vi "Senden_ECD.vi"(5 "error in":errorcluster, 6 "BefehlsCluster":T1, 7 "AbfragenCluster":cluster{string[], string[], string[]}, 8 "Abfragenr.Cluster":cluster{i32, i32, i32}, 9 "Senden?":bool[](array[boolean]), 10 "FPGA-VI-Referenz":refnum<k20>) -> (0 "BefehlsCluster":T1, 2 "error out":errorcluster, 3 "Senden?":bool[](array[boolean]), 4 "Abfragenr.Cluster":cluster{i32, i32, i32})   [LabVIEW 2017]
uses:
  <vilib>/Utility/error.llb/Error Cluster From Error Code.vi
  <vilib>/rvi/errors/niLvFpgaAdjustHostInterfaceError.vi
  <vilib>/rvi/interface/nirviMethod/nirviMethod.xnode
  FPGA Bitfiles/HAGAR-VECD_FPGATarget_FPGA-ProgrammECD_WS++LmW9gGg.lvbitx
  FPGA-Programm_ECD.vi
  <vilib>/rvi/errors/niLvFpgaMergeErrorWithErrorCode.vi
  <vilib>/FPGAPlugInAG/cRIO-9035/niLvFpga_WriteFifo_cRIO-9035.vi
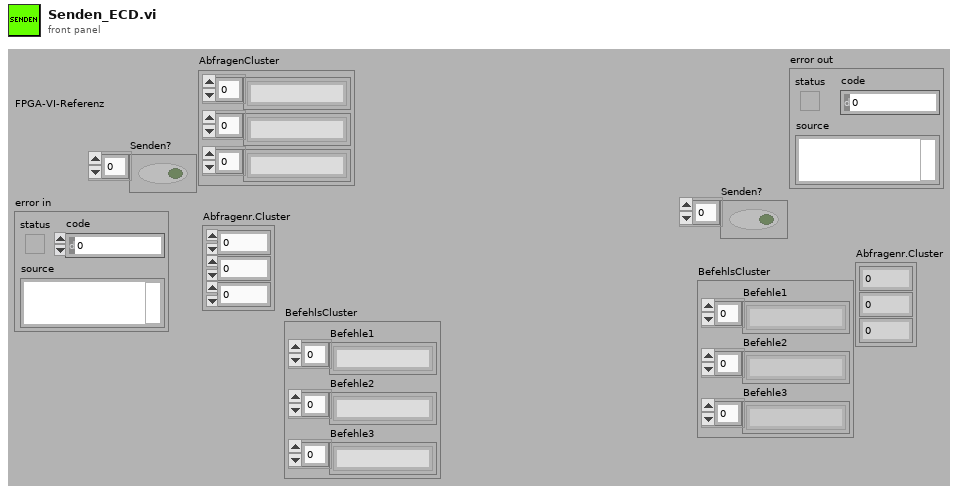
[diagram p1: front panel]
types:
  T1 = cluster{"Befehle1":string[], "Befehle2":string[], "Befehle3":string[]}
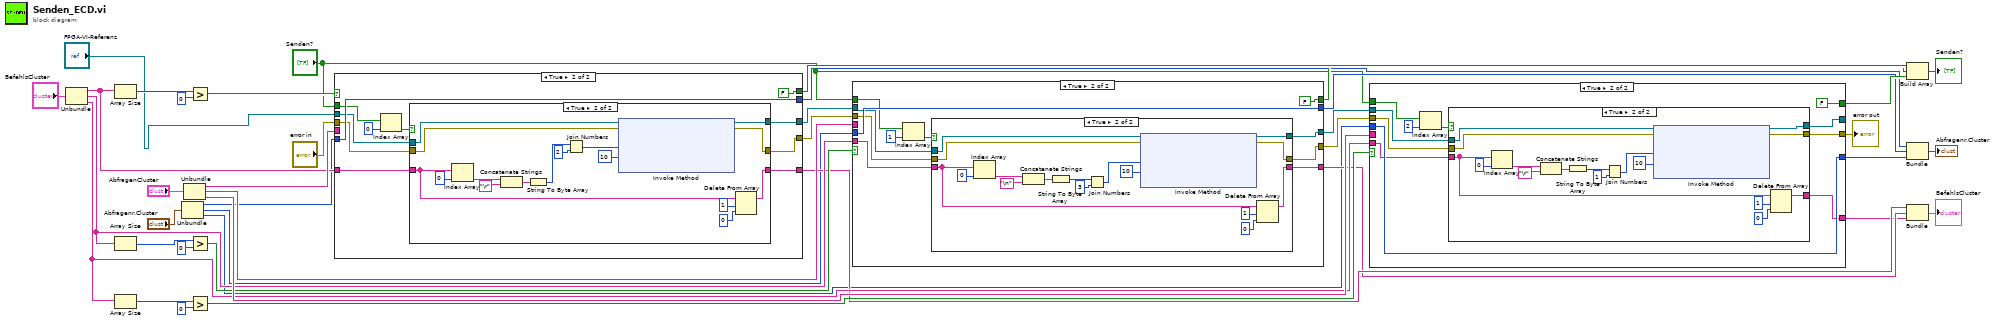
[diagram p0: block diagram]
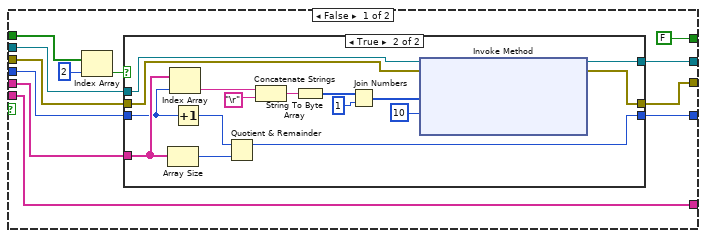
[diagram p2: hidden frame]
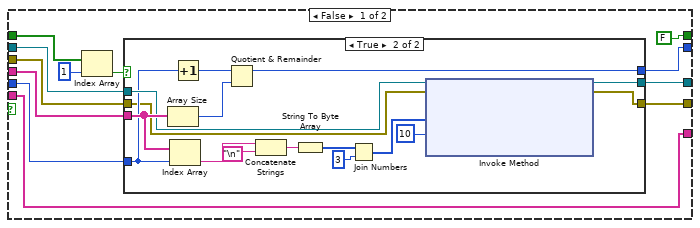
[diagram p5: hidden frame]
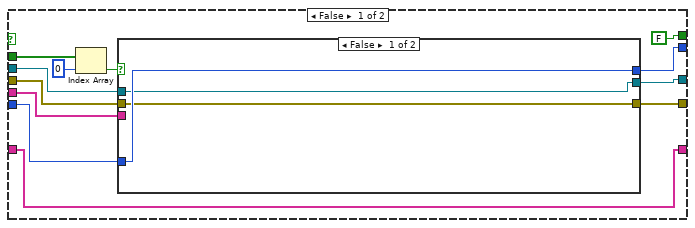
[diagram p8: hidden frame]
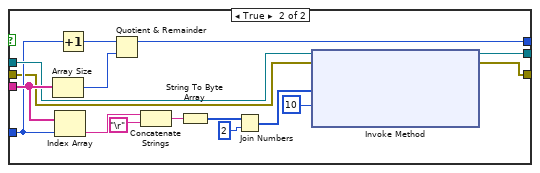
[diagram p9: hidden frame]
diagram:
  n1 = Unbundle("BefehlsCluster") -> ("Befehle1"=w26:string[], "Befehle2"=w25:string[], "Befehle3"=w24:string[])
  n2 = Array Size(array=w26) -> (size(s)=w41:i32)
  n3 = Array Size(array=w25) -> (size(s)=w35:i32)
  n4 = Array Size(array=w24) -> (size(s)=w32:i32)
  n5 = Unbundle("Abfragenr.Cluster") -> (w14:i32, w13:i32, w12:i32)
  n6 = Unbundle("AbfragenCluster") -> (w38:string[], w37:string[], w36:string[])
  n7 = Greater?(x=w41, y=0) -> (0:w39:bool)
  n8 = Greater?(x=w35, y=0) -> (0:w33:bool)
  n9 = Greater?(x=w32, y=0) -> (0:w30:bool)
  n10 = case shown="True" w39 {
    tunnel: w26 -> [w53 w80]
    tunnel: [w53 w79] -> w23
    tunnel: "Senden?" -> [w47 w77]
    tunnel: [FALSE FALSE] -> w19
    tunnel: w14 -> [w50 w83]
    tunnel: "FPGA-VI-Referenz" -> [w49 w78]
    tunnel: [w48 w83] -> w11
    tunnel: w38 -> [w46 _]
    tunnel: [w45 w76] -> w29
    tunnel: "error in" -> [w43 w74]
    tunnel: [w42 w73] -> w4
    frame False {
      n11 = Index Array(array=w47, index=0 ("Index")) -> (element=w51:bool)
      n12 = case shown="False" w51 {
        tunnel: w46 -> [_ w70]
        tunnel: w50 -> [w56 w64]
        tunnel: w49 -> [w55 w67]
        tunnel: [w56 w63] -> w48
        tunnel: [w55 w62] -> w45
        tunnel: w43 -> [w54 w58]
        tunnel: [w54 w57] -> w42
        frame False {
        }
        frame True {
          n13 = Array Size(array=w70) -> (size(s)=w71:i32)
          n14 = Index Array(array=w70, index=w64) -> (element=w60:string)
          n15 = Increment(x=w64) -> (x+1=w72:i32)
          n16 = Quotient & Remainder(x=w72, y=w71) -> (x-y*floor(x/y)=w63:i32)  [unwired: 1 out]
          n17 = Concatenate Strings(w60, "\r") -> (w61:string)
          n18 = String To Byte Array(string=w61) -> (unsigned byte array=w69:u8[])
          n19 = Join Numbers(hi=w69, lo=u8 2) -> ((hi.lo)=w66:u16[])
          n20 = xnode "Invoke Method"("FPGA-VI-Referenz (Eingang)"=w67, "Fehler (Eingang)"=w58, "Daten"=w66, "Timeout (ms)"=10) -> ("FPGA-VI-Referenz (Ausgang)"=w62:refnum<k20>, "Fehler (Ausgang)"=w57:errorcluster)  [unwired: 1 out]
        }
      }
    }
    frame True {
      n21 = Index Array(array=w77, index=0 ("Index")) -> (element=w81:bool)
      n22 = case shown="True" w81 {
        tunnel: w80 -> [w86 w98]
        tunnel: [w86 w100] -> w79
        tunnel: w78 -> [w85 w99]
        tunnel: [w85 w92] -> w76
        tunnel: w74 -> [w84 w88]
        tunnel: [w84 w87] -> w73
        frame False {
        }
        frame True {
          n23 = Index Array(array=w98, index=0 ("Index")) -> (element=w90:string)
          n24 = Concatenate Strings(w90, "\r") -> (w89:string)
          n25 = String To Byte Array(string=w89) -> (unsigned byte array=w96:u8[])
          n26 = Join Numbers(hi=w96, lo=u8 2) -> ((hi.lo)=w94:u16[])
          n27 = xnode "Invoke Method"("FPGA-VI-Referenz (Eingang)"=w99, "Fehler (Eingang)"=w88, "Daten"=w94, "Timeout (ms)"=10) -> ("FPGA-VI-Referenz (Ausgang)"=w92:refnum<k20>, "Fehler (Ausgang)"=w87:errorcluster)  [unwired: 1 out]
          n28 = Delete From Array(array=w98, length=1 ("Länge"), index=0 ("Index")) -> (array with subset deleted=w100:string[])  [unwired: 1 out]
        }
      }
    }
  }
  n29 = case shown="True" w33 {
    tunnel: w25 -> [w114 w141]
    tunnel: [w114 w140] -> w22
    tunnel: "Senden?" -> [w108 w138]
    tunnel: w13 -> [w111 w144]
    tunnel: w29 -> [w110 w139]
    tunnel: [w109 w144] -> w10
    tunnel: w37 -> [w107 _]
    tunnel: [w106 w137] -> w28
    tunnel: [FALSE FALSE] -> w17
    tunnel: w4 -> [w104 w135]
    tunnel: [w103 w134] -> w3
    frame False {
      n30 = Index Array(array=w108, index=1 ("Index")) -> (element=w112:bool)
      n31 = case shown="True" w112 {
        tunnel: w107 -> [_ w131]
        tunnel: w111 -> [w117 w125]
        tunnel: w110 -> [w116 w128]
        tunnel: [w117 w124] -> w109
        tunnel: [w116 w123] -> w106
        tunnel: w104 -> [w115 w119]
        tunnel: [w115 w118] -> w103
        frame False {
        }
        frame True {
          n32 = Array Size(array=w131) -> (size(s)=w132:i32)
          n33 = Index Array(array=w131, index=w125) -> (element=w121:string)
          n34 = Increment(x=w125) -> (x+1=w133:i32)
          n35 = Quotient & Remainder(x=w133, y=w132) -> (x-y*floor(x/y)=w124:i32)  [unwired: 1 out]
          n36 = Concatenate Strings(w121, "\n") -> (w120:string)
          n37 = String To Byte Array(string=w120) -> (unsigned byte array=w130:u8[])
          n38 = Join Numbers(hi=w130, lo=u8 3) -> ((hi.lo)=w127:u16[])
          n39 = xnode "Invoke Method"("FPGA-VI-Referenz (Eingang)"=w128, "Fehler (Eingang)"=w119, "Daten"=w127, "Timeout (ms)"=10) -> ("FPGA-VI-Referenz (Ausgang)"=w123:refnum<k20>, "Fehler (Ausgang)"=w118:errorcluster)  [unwired: 1 out]
        }
      }
    }
    frame True {
      n40 = Index Array(array=w138, index=1 ("Index")) -> (element=w142:bool)
      n41 = case shown="True" w142 {
        tunnel: w141 -> [w147 w159]
        tunnel: [w147 w161] -> w140
        tunnel: w139 -> [w146 w160]
        tunnel: [w146 w153] -> w137
        tunnel: w135 -> [w145 w149]
        tunnel: [w145 w148] -> w134
        frame False {
        }
        frame True {
          n42 = Index Array(array=w159, index=0 ("Index")) -> (element=w151:string)
          n43 = Concatenate Strings(w151, "\n") -> (w150:string)
          n44 = String To Byte Array(string=w150) -> (unsigned byte array=w157:u8[])
          n45 = Join Numbers(hi=w157, lo=u8 3) -> ((hi.lo)=w155:u16[])
          n46 = xnode "Invoke Method"("FPGA-VI-Referenz (Eingang)"=w160, "Fehler (Eingang)"=w149, "Daten"=w155, "Timeout (ms)"=10) -> ("FPGA-VI-Referenz (Ausgang)"=w153:refnum<k20>, "Fehler (Ausgang)"=w148:errorcluster)  [unwired: 1 out]
          n47 = Delete From Array(array=w159, length=1 ("Länge"), index=0 ("Index")) -> (array with subset deleted=w161:string[])  [unwired: 1 out]
        }
      }
    }
  }
  n48 = case shown="True" w30 {
    tunnel: w24 -> [w175 w202]
    tunnel: [w175 w201] -> w21
    tunnel: "Senden?" -> [w169 w199]
    tunnel: w12 -> [w172 w205]
    tunnel: w28 -> [w171 w200]
    tunnel: [w170 w205] -> w9
    tunnel: w36 -> [w168 _]
    tunnel: [FALSE FALSE] -> w16
    tunnel: [w166 w197] -> _
    tunnel: w3 -> [w165 w196]
    tunnel: [w164 w195] -> w2
    frame False {
      n49 = Index Array(array=w169, index=2 ("Index")) -> (element=w173:bool)
      n50 = case shown="True" w173 {
        tunnel: w168 -> [_ w192]
        tunnel: w172 -> [w178 w186]
        tunnel: w171 -> [w177 w189]
        tunnel: [w178 w185] -> w170
        tunnel: [w177 w184] -> w166
        tunnel: w165 -> [w176 w180]
        tunnel: [w176 w179] -> w164
        frame False {
        }
        frame True {
          n51 = Array Size(array=w192) -> (size(s)=w193:i32)
          n52 = Index Array(array=w192, index=w186) -> (element=w182:string)
          n53 = Increment(x=w186) -> (x+1=w194:i32)
          n54 = Quotient & Remainder(x=w194, y=w193) -> (x-y*floor(x/y)=w185:i32)  [unwired: 1 out]
          n55 = Concatenate Strings(w182, "\r") -> (w181:string)
          n56 = String To Byte Array(string=w181) -> (unsigned byte array=w191:u8[])
          n57 = Join Numbers(hi=w191, lo=u8 1) -> ((hi.lo)=w188:u16[])
          n58 = xnode "Invoke Method"("FPGA-VI-Referenz (Eingang)"=w189, "Fehler (Eingang)"=w180, "Daten"=w188, "Timeout (ms)"=10) -> ("FPGA-VI-Referenz (Ausgang)"=w184:refnum<k20>, "Fehler (Ausgang)"=w179:errorcluster)  [unwired: 1 out]
        }
      }
    }
    frame True {
      n59 = Index Array(array=w199, index=2 ("Index")) -> (element=w203:bool)
      n60 = case shown="True" w203 {
        tunnel: w202 -> [w208 w220]
        tunnel: [w208 w222] -> w201
        tunnel: w200 -> [w207 w221]
        tunnel: [w207 w214] -> w197
        tunnel: w196 -> [w206 w210]
        tunnel: [w206 w209] -> w195
        frame False {
        }
        frame True {
          n61 = Index Array(array=w220, index=0 ("Index")) -> (element=w212:string)
          n62 = Concatenate Strings(w212, "\r") -> (w211:string)
          n63 = String To Byte Array(string=w211) -> (unsigned byte array=w218:u8[])
          n64 = Join Numbers(hi=w218, lo=u8 1) -> ((hi.lo)=w216:u16[])
          n65 = xnode "Invoke Method"("FPGA-VI-Referenz (Eingang)"=w221, "Fehler (Eingang)"=w210, "Daten"=w216, "Timeout (ms)"=10) -> ("FPGA-VI-Referenz (Ausgang)"=w214:refnum<k20>, "Fehler (Ausgang)"=w209:errorcluster)  [unwired: 1 out]
          n66 = Delete From Array(array=w220, length=1 ("Länge"), index=0 ("Index")) -> (array with subset deleted=w222:string[])  [unwired: 1 out]
        }
      }
    }
  }
  "error out" <- w2
  n67 = Build Array(w19, w17, w16) -> (→"Senden?":bool[])
  n68 = Bundle(w11, w10, w9) -> (→"Abfragenr.Cluster":cluster{i32, i32, i32})  [unwired: 1 in]
  n69 = Bundle("Befehle1"=w23, "Befehle2"=w22, "Befehle3"=w21) -> (→"BefehlsCluster":T1)  [unwired: 1 in]
